vi "F Dwf Device Param Get.vi"(8 "error in (no error)":errorcluster, 9 "pvalue":i32, 10 "param":i32, 11 "hdwf":i32) -> (0 "error out":errorcluster, 1 "pvalue out":i32, 3 "function return":i32)   [LabVIEW 2021, in "Olasdwf.lvlib"]
doc: "DWFAPI int FDwfDeviceParamGet(HDWF hdwf, DwfParam param, int *pvalue);"
uses:
  Olasdwf.lvlib
  Windows/System32/dwf.dll
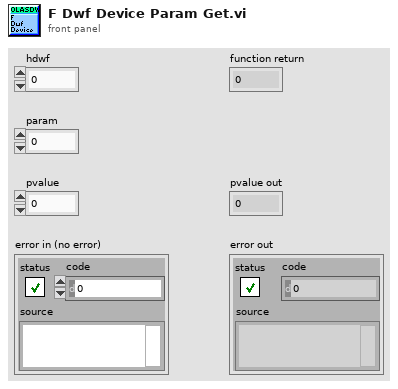
[diagram p1: front panel]
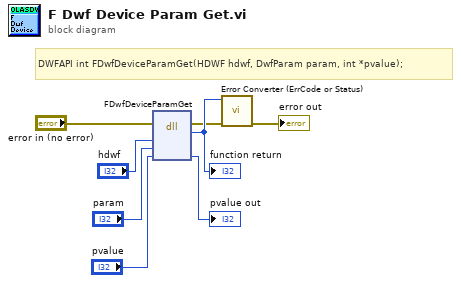
[diagram p0: block diagram]
diagram:
  # "DWFAPI int FDwfDeviceParamGet(HDWF hdwf, DwfParam param, int *pvalue);"
  n1 = dll-call lib="/Windows/System32/dwf.*" fn="FDwfDeviceParamGet"(error in="error in (no error)", "hdwf"="hdwf", "param"="param", "pvalue"="pvalue") -> (error out=w2:errorcluster, w8:i32, "pvalue"=→"pvalue out":i32)  [unwired: 4 in, 1 out]
  "function return" <- w8
  n2 = call "Error Converter (ErrCode or Status).vi"("error in (no error)"=w2, "error code"=w8) -> ("error out"=→"error out":errorcluster)  [unwired: 9 in]
